vi "VI Tester Add Test To TestCase.vi"(8 "error in":errorcluster, 10 "Active VI Info":T1, 11 "TestCase Refnum":refnum<vi>) -> (0 "error out":errorcluster)   [LabVIEW 2009]
uses:
  <vilib>/addons/_JKI Toolkits/RCF API/Right Click API.llb/Framework - Active VI Info - Cluster - __RightClickAPI.ctl
  <vilib>/addons/_JKI Toolkits/RCF API/Right Click API.llb/Framework - Selection Type - Enum - __RightClickAPI.ctl
  <vilib>/addons/_JKI Toolkits/RCF API/Right Click API.llb/RightClickAPI.lvlib
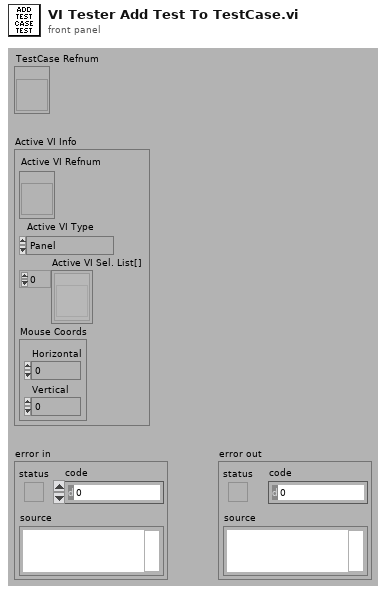
[diagram p1: front panel]
types:
  T1 = typedef "RightClickAPI.lvlib/Framework - Active VI Info - Cluster - __RightClickAPI.ctl" = cluster{"Active VI Refnum":refnum<vi>, "Active VI Type":T2, "Active VI Sel. List[]":refnum<vi>[], "Mouse Coords":cluster{"Horizontal":i32, "Vertical":i32}}
  T2 = typedef "RightClickAPI.lvlib/Framework - Selection Type - Enum - __RightClickAPI.ctl" = enum16{"Panel", "Diagram"}
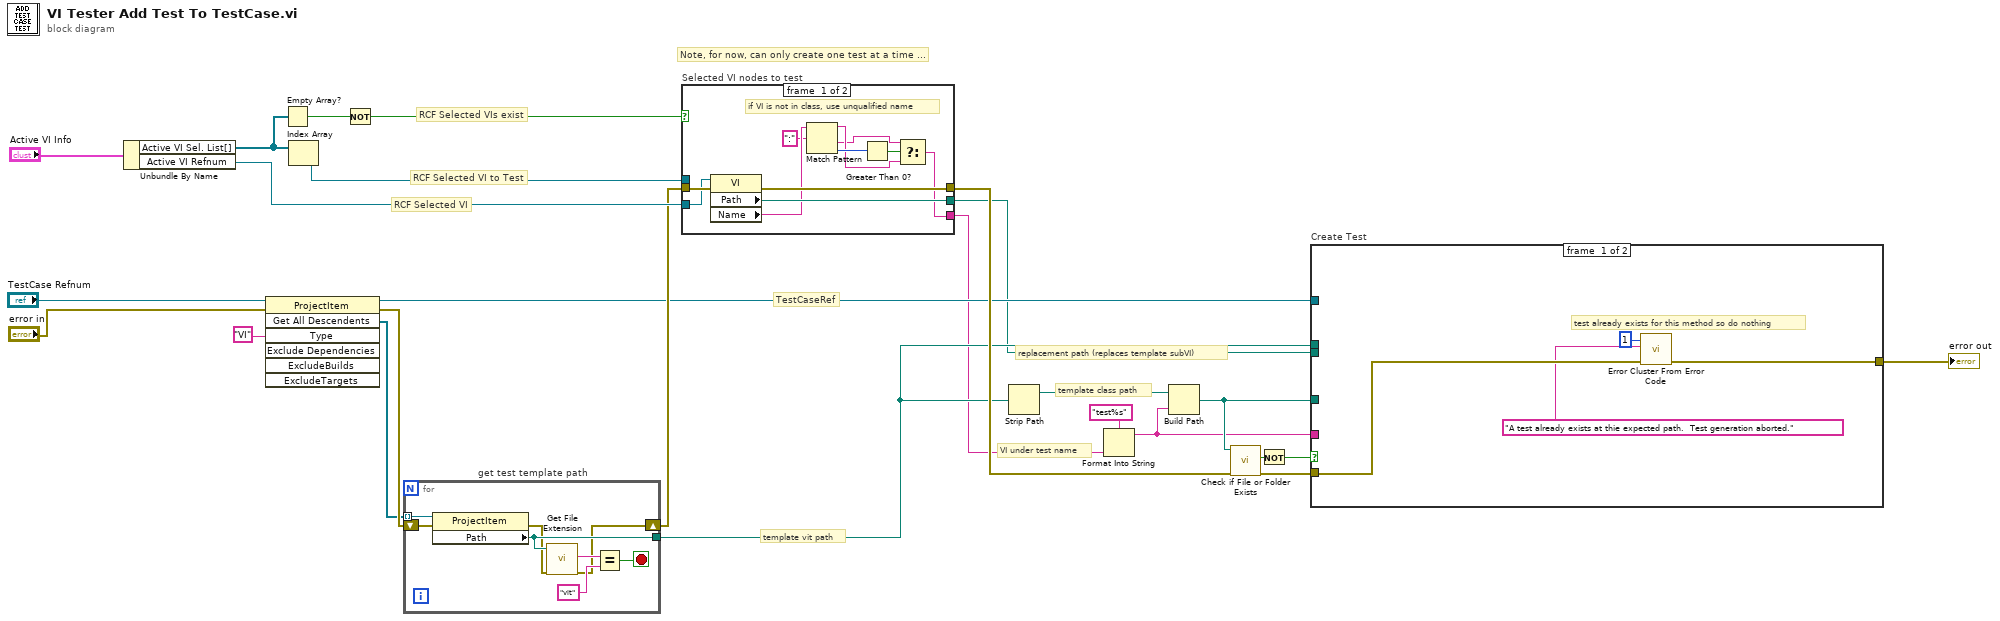
[diagram p0: block diagram]
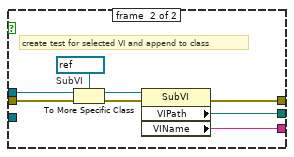
[diagram p2: hidden frame]
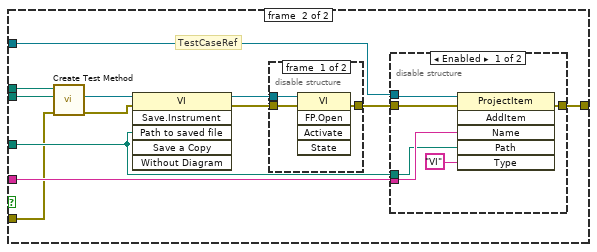
[diagram p3: hidden frame]
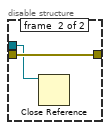
[diagram p4: hidden frame]
diagram:
  # "VI under test name"
  # "Note, for now, can only create one test at a time ..."
  # "RCF Selected VIs exist"
  # "RCF Selected VI"
  # "RCF Selected VI to Test"
  # "replacement path (replaces template subVI)"
  # "template class path"
  # "TestCaseRef"
  # "template vit path"
  n1 = Unbundle By Name("Active VI Info") -> ("Active VI Sel. List[]"=w20:refnum<vi>[], "Active VI Refnum"=w25:refnum<vi>)
  n2 = invoke class="ProjectItem" method="Get All Descendents"(reference="TestCase Refnum", error in="error in", "Type"="VI") -> (reference out=w17:refnum<vi>, error out=w6:errorcluster, "All Descendents"=w5:refnum<vi>[])  [unwired: 4 in, 4 out]
  n3 = Empty Array?(array=w20) -> (empty?=w22:bool)
  n4 = Index Array(array=w20) -> (element=w3:refnum<vi>)  [unwired: 1 in]
  n5 = Not(x=w22) -> (.not. x?=w1:bool)
  n6 = for "get test template path" {
    tunnel: w5 -> [w33] mode=indexing
    tunnel: [w29] -> w16
    shift-right: [w26] -> w21
    shift-left: w6 -> [w28]
    stop <- w30 stop-if-true
    n7 = property class="ProjectItem"(reference=w33, error in=w28) -> (error out=w27:errorcluster, "Path"=w29:path)  [unwired: 1 out]
    n8 = call <vilib>:"Get File Extension.vi"("error in (no error)"=w27, "file"=w29) -> ("error out"=w26:errorcluster, "lowercase file extension"=w32:string)  [unwired: 6 in, 2 out]
    n9 = Equal?(x=w32, y="vit") -> (x = y?=w30:bool)
  }
  n10 = case "Selected VI nodes to test" shown="False" w1 {
    tunnel: w3 -> [_ w52]
    tunnel: [w34 w49] -> w14
    tunnel: [w44 w48] -> w15
    tunnel: [w43 w47] -> w18
    tunnel: w21 -> [w42 w46]
    tunnel: w25 -> [w41 _]
    frame #0 {
      # "if VI is not in class, use unqualified name"
      n11 = property class="VI"(reference=w41, error in=w42) -> (error out=w43:errorcluster, "Path"=w44:path, "Name"=w40:string)  [unwired: 1 out]
      n12 = Match Pattern(string=w40, regular expression=":") -> (before substring=w36:string, after substring=w35:string, offset past match=w38:i32)  [unwired: 1 in, 1 out]
      n13 = Greater Than 0?(x=w38) -> (x > 0?=w37:bool)
      n14 = Select(t=w35, s=w37, f=w36) -> (s? t:f=w34:string)
    }
    frame #1 {
      w51 = refnum<vi> refnum  # SubVI
      # "create test for selected VI and append to class"
      n15 = To More Specific Class(target class=w51, reference=w52, error in=w46) -> (specific class reference=w50:refnum<vi>, error out=w45:errorcluster)
      n16 = property class="SubVI"(reference=w50, error in=w45) -> (error out=w47:errorcluster, "VIPath"=w48:path, "VIName"=w49:string)  [unwired: 1 out]
    }
  }
  n17 = Strip Path(path=w16) -> (stripped path=w23:path)  [unwired: 1 out]
  n18 = Format Into String(format string="test%s", w14) -> (resulting string=w9:string)  [unwired: 2 in, 1 out]
  n19 = Build Path(base path=w23, name or relative path=w9) -> (appended path=w10:path)
  n20 = call <vilib>:"Check if File or Folder Exists.vi"("error in (no error)"=w18, "path"=w10) -> ("error out"=w11:errorcluster, "file or folder exists?"=w12:bool)  [unwired: 7 in, 1 out]
  n21 = Not(x=w12) -> (.not. x?=w13:bool)
  n22 = case "Create Test" shown="False" w13 {
    tunnel: w16 -> [_ w68]
    tunnel: w17 -> [_ w67]
    tunnel: w9 -> [_ w65]
    tunnel: [w55 w64] -> w19
    tunnel: w15 -> [_ w63]
    tunnel: w10 -> [_ w61]
    tunnel: w11 -> [w56 w60]
    frame #0 {
      # "test already exists for this method so do nothing"
      n23 = call <vilib>:"Error Cluster From Error Code.vi"("error in (no error)"=w56, "error message (\"\")"="A test already exists at thie expected path.  Test generation aborted." ("error message (\"\")"), "error code (0)"=1) -> ("error out"=w55:errorcluster)  [unwired: 6 in]
    }
    frame #1 {
      # "TestCaseRef"
      n24 = call "Create Test Method.vi"("error in"=w60, "Replacement VI"=w63, "template test VI"=w68) -> ("error out"=w62:errorcluster, "New VI Refnum"=w66:refnum<vi>)  [unwired: 7 in]
      n25 = invoke class="VI" method="Save.Instrument"(reference=w66, error in=w62, "Path to saved file"=w61) -> (reference out=w59:refnum<vi>, error out=w58:errorcluster)  [unwired: 3 in, 4 out]
      n26 = disable-structure shown="Enabled" {
        disable-tunnel: w59 -> [w71 w72]
        disable-tunnel: w58 -> [w70 w73]
        disable-tunnel: [w69 w73] -> w57
        frame #0 {
          n27 = invoke class="VI" method="FP.Open"(reference=w71, error in=w70) -> (error out=w69:errorcluster)  [unwired: 3 in, 4 out]
        }
        frame #1 {
          n28 = Close Reference(reference=w72) -> ()  [unwired: 1 in, 1 out]
        }
      }
      n29 = disable-structure shown="Enabled" {
        disable-tunnel: w67 -> [w78 _]
        disable-tunnel: w65 -> [w77 _]
        disable-tunnel: [w76 w80] -> w64
        disable-tunnel: w61 -> [w75 _]
        disable-tunnel: w57 -> [w74 w80]
        frame #0 {
          n30 = invoke class="ProjectItem" method="AddItem"(reference=w78, error in=w74, "Name"=w77, "Path"=w75, "Type"="VI") -> (error out=w76:errorcluster)  [unwired: 1 in, 5 out]
        }
        frame #1 {
          # "can't add method because class\nis locked"
        }
      }
    }
  }
  "error out" <- w19
